vi "TFG.vi"() -> ()   [LabVIEW 2023]
uses:
  C:/Program Files (x86)/National Instruments/LabVIEW 2023/examples/Instrument IO/Serial/support/Serial - Settings.ctl
  <vilib>/Analysis/3filter.llb/Filter Passband Type.ctl
  <vilib>/Waveform/WDTOps.llb/WDT Waveform Duration DBL.vi
  <vilib>/Waveform/WDTOps.llb/WDT Number of Waveform Samples DBL.vi
  <vilib>/Waveform/WDTOps.llb/WDT Get Waveform Subset DBL.vi
  <vilib>/Analysis/3filter.llb/Butterworth Filter (DBL).vi
  <vilib>/measure/mamon.llb/Waveform Peak Detection for 1 Chan.vi
  <vilib>/express/express analysis/Spectral/Block/exnSpectralBlock spectral measurements power poly.vi
  <vilib>/express/express analysis/Spectral/Block/exnSpectralBlock spectral measurements power WFM.vi
  <vilib>/Instr/_visa.llb/VISA Configure Serial Port (Instr).vi
  <vilib>/express/express analysis/Spectral/XNode/ExpressSpectralMeasurementsBlockNode.xnode
  <vilib>/Analysis/NI_AALBase.lvlib
  <vilib>/measure/NI_MAPro.lvlib
  <vilib>/Analysis/NI_AALPro.lvlib
panel:
  in  "End Write on Termination Character? 2":bool=TRUE
  in  "Serial Settings (write) 2":T1={"baud rate"=9600, "data bits"=8, "parity"=enum."None", "stop bits"=10, "flow control"=0} {"flow control" items=["None"=0, "XON/XOFF"=1, "RTS/CTS"=2, "DTR/DSR"=4]; "stop bits" items=["1.0"=10, "1.5"=15, "2.0"=20]; "data bits" min=5 max=8 step=1; "baud rate" items=["75"=75, "110"=110, "134"=134, "150"=150, "300"=300, "600"=600, "1200"=1200, "1800"=1800, "2400"=2400, "4800"=4800, "7200"=7200, "9600"=9600, "14400"=14400, "19200"=19200, "28800"=28800, "38400"=38400, "56000"=56000, "57600"=57600, "115200"=115200, "128000"=128000, "230400"=230400]}
  in  "VISA Resource (write) 2":refnum<visa-resource-name>="COM1"
  out "bytes written 2":u32
  out "Formas de onda":waveform(dbl)[](graph)
  out "Señal Adquirida 2":waveform(dbl)[](graph)
  out "frecuencia manual 3":string
  out "frecuencia manual 1":string
  in  "banda 2":dbl
  in  "banda 1":dbl
  in  "peaks/valleys 2":u16(ring) items=["Peaks", "Valleys"]
  in  "duration":dbl=1.0 format="%0.2f"
  in  "alpha":dbl
  in  "path":path
  in  "Apagado":bool
  out "Baja con filtro":dbl
  out "baja sin filtro":dbl
  in  "Frecuencia manual1":dbl(slide) scale=150.0..3000.0
  in  "frecuencia manual 2":dbl(slide) scale=150.0..3000.0
  out "Espectro Amplitud":cluster{"f0":dbl, "df":dbl, "magnitude":dbl[]}(graph)
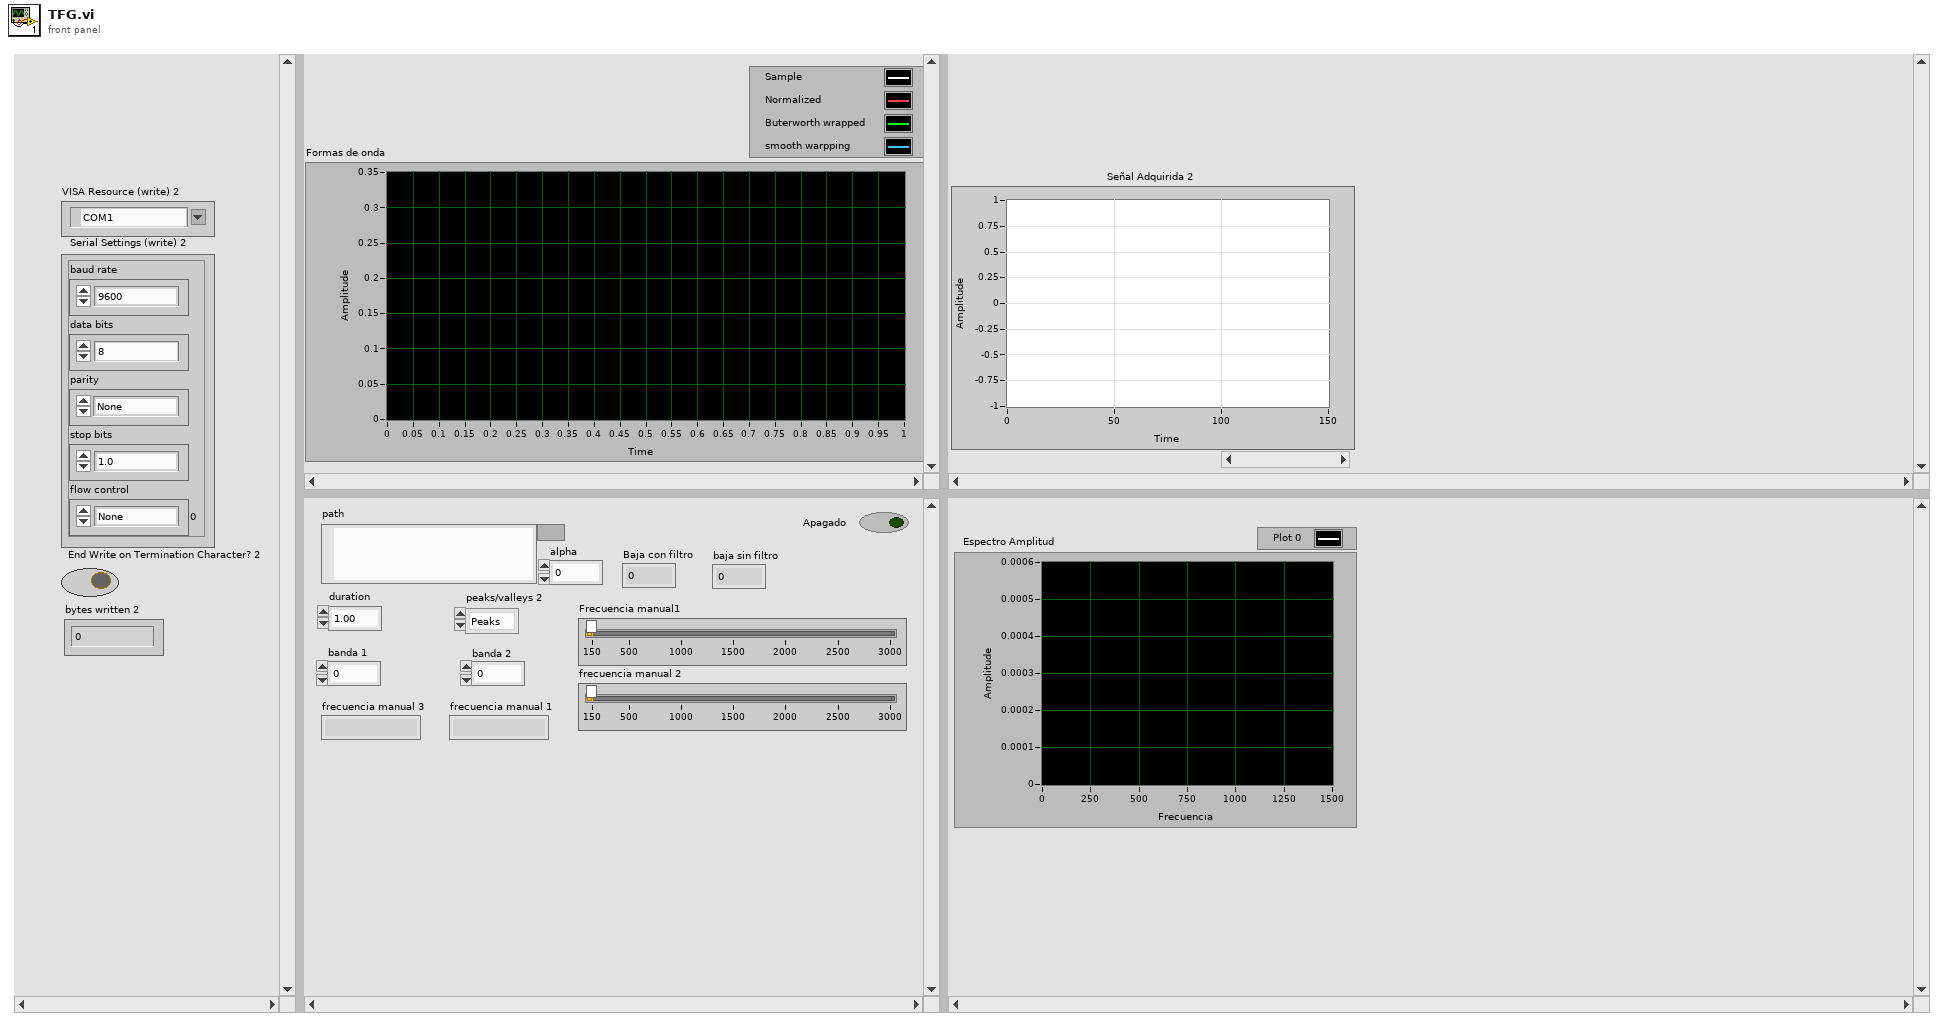
[diagram p1: front panel]
types:
  T1 = typedef "Serial - Settings.ctl" = cluster{"baud rate":u32, "data bits":u16, "parity":enum16{"None", "Odd", "Even", "Mark", "Space"}, "stop bits":u16, "flow control":u16}
  T2 = typedef "NI_AALBase.lvlib/Filter Passband Type.ctl" = enum32{"Lowpass", "Highpass", "Bandpass", "Bandstop"}
  T3 = cluster{"averaging mode":u16, "weighting mode":u16, "number of averages":u32}
  T4 = cluster{"dB On (F)":bool, "unwrap phase (F)":bool, "convert to degree (F)":bool}
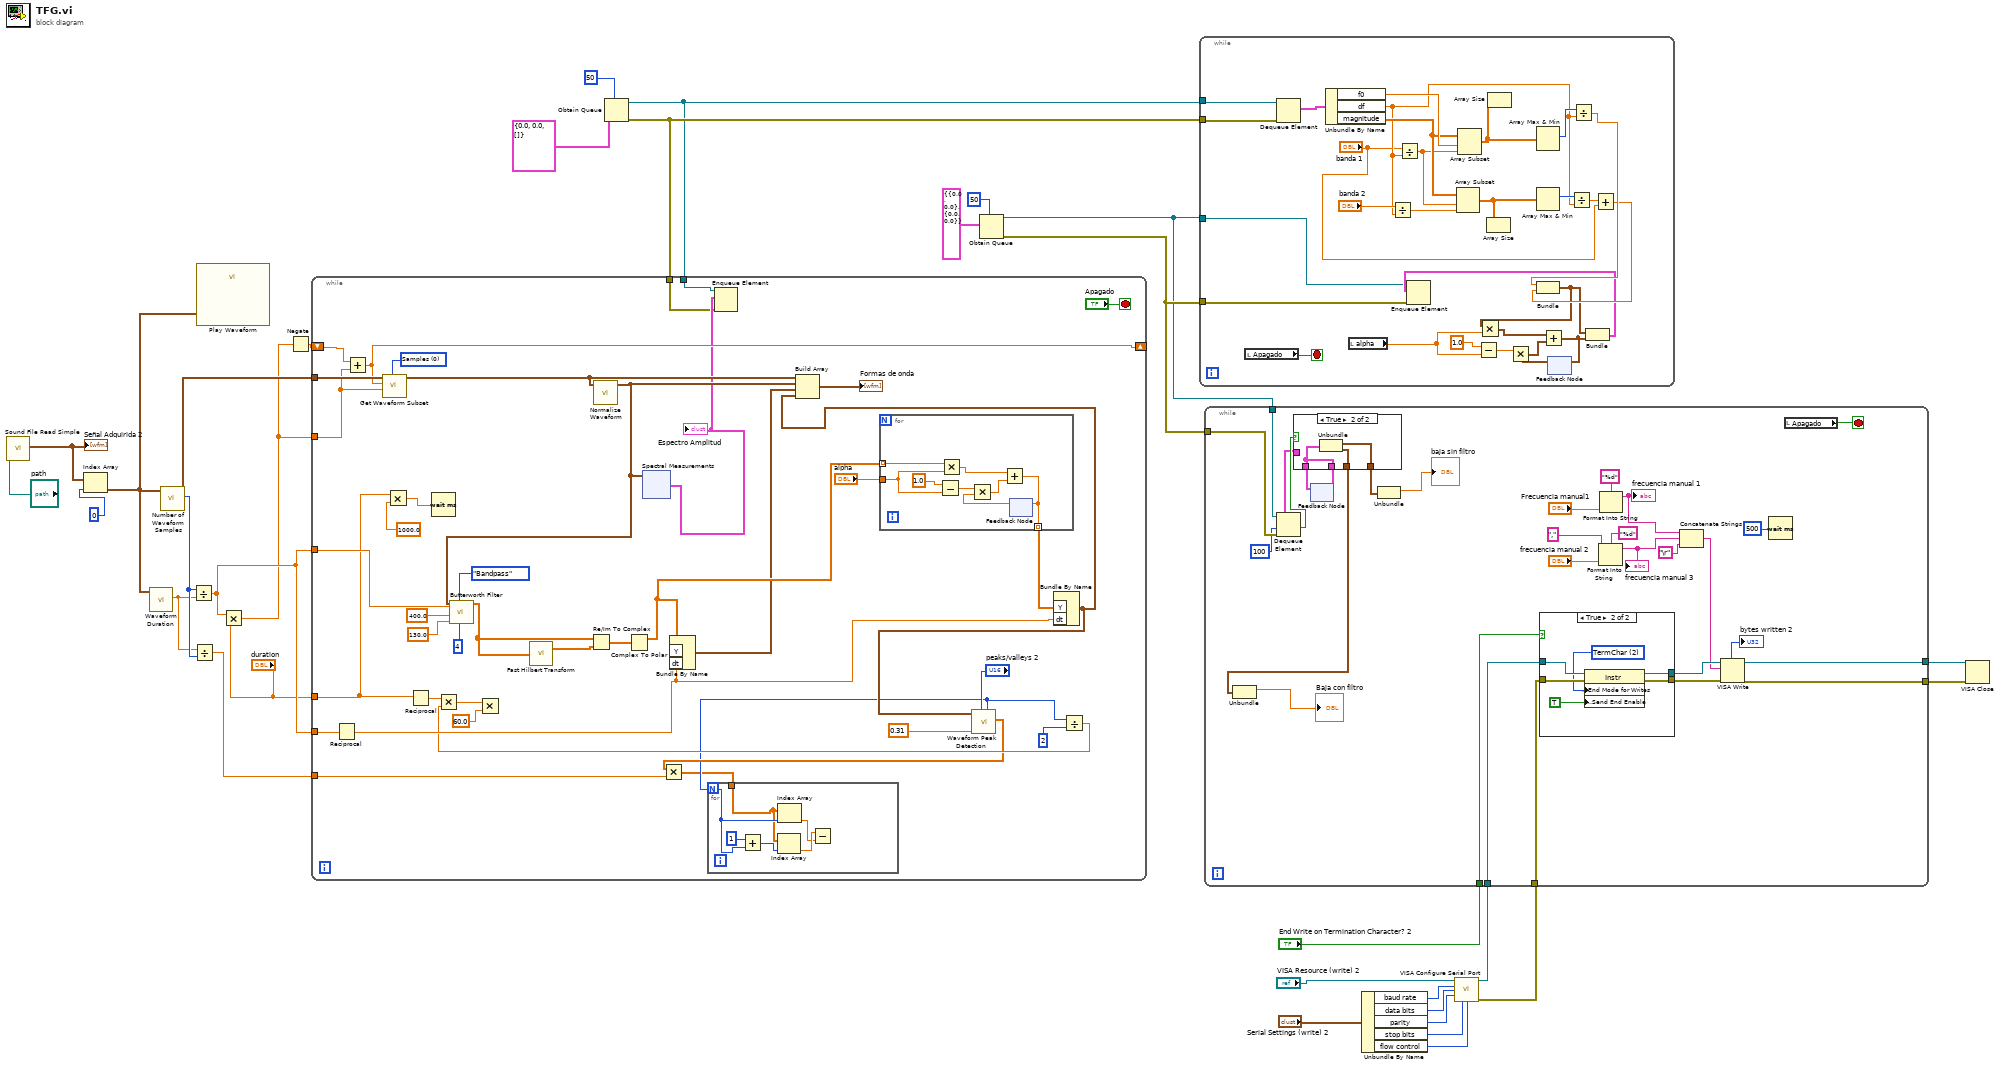
[diagram p0: block diagram]
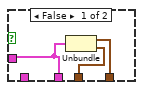
[diagram p3: hidden frame]
diagram:
  n1 = call <vilib>:"Sound File Read Simple.vi"("path"="path") -> ("data"=w31:waveform(dbl)[])  [unwired: 7 in, 3 out]
  "Señal Adquirida 2" <- w31
  n2 = Index Array(array=w31, index=0) -> (element=w22:waveform(dbl))
  n3 = call-poly <vilib>:"Waveform Duration.vi"("waveform in"=w22) -> ("duration"=w27:dbl)  [unwired: 8 in, 2 out]
  n4 = call-poly <vilib>:"Number of Waveform Samples.vi"("waveform in"=w22) -> ("number of samples"=w29:i32, "waveform out"=w28:waveform(dbl))  [unwired: 8 in, 1 out]
  n5 = Divide(x=w29, y=w27) -> (x/y=w25:dbl)
  n6 = Divide(x=w27, y=w29) -> (x/y=w26:dbl)
  n7 = call "Play Waveform"("Data"=w22) -> ()  [unwired: 18 in, 1 out]
  n8 = Multiply(x=w25, y="duration") -> (x*y=w24:dbl)
  n9 = Negate(x=w24) -> (-x=w23:dbl)
  n10 = Obtain Queue(max queue size (-1, unlimited)=50, element data type=cluster{"f0":dbl, "df":dbl, "magnitude":dbl[]} {"f0"=0.0, "df"=0.0, "magnitude"=[]} ("Power Spectrum")) -> (queue out=w16:refnum<queue>, error out=w19:errorcluster)  [unwired: 3 in, 1 out]
  n11 = while {
    tunnel: w28 -> [w47]
    tunnel: w26 -> [w46]
    tunnel: w25 -> [w45]
    shift-right: [w37] -> _
    shift-left: w23 -> [w38]
    tunnel: w25 -> [w41]
    tunnel: "duration" -> [w40]
    tunnel: w24 -> [w39]
    tunnel: w19 -> [w34]
    tunnel: w16 -> [w33]
    stop <- "Apagado" stop-if-true
    w42 = u16 0 items=["Samples", "Relative Time"] ("start/duration format")
    n12 = Reciprocal(x=w41) -> (1/x=w57:dbl)
    n13 = Add(x=w38, y=w39) -> (x+y=w37:dbl)
    n14 = call-poly <vilib>:"Get Waveform Subset.vi"("start/duration format"=w42, "duration"=w39, "start samples/time"=w37, "waveform in"=w47) -> ("waveform out"=w36:waveform(dbl))  [unwired: 2 in, 3 out]
    n15 = Multiply(x=w40, y=1000.0) -> (x*y=w44:dbl)
    n16 = Reciprocal(x=w40) -> (1/x=w54:dbl)
    n17 = Wait (ms)(milliseconds to wait=w44) -> ()  [unwired: 1 out]
    n18 = call <vilib>:"Normalize Waveform.vi"("waveform in"=w36) -> ("normalized waveform"=w68:waveform(dbl))  [unwired: 7 in, 3 out]
    n19 = call-poly <vilib>:"Butterworth Filter.vi"("order"=4, "filter type"=Filter_Passband_Type."Bandpass", "low cutoff freq: fl"=130.0, "high cutoff freq: fh"=400.0 ("low cutoff freq: fl"), "sampling freq: fs"=w45, "X"=w68) -> ("Filtered X"=w63:dbl[])  [unwired: 2 in, 1 out]
    n20 = call <vilib>:"Fast Hilbert Transform.vi"("X"=w63) -> ("Hilbert{X}"=w64:dbl[])  [unwired: 1 out]
    n21 = Re/Im To Complex(1:w64, 2:w63) -> (0:w62:cdb[])
    n22 = Complex To Polar(r * e^(i*theta)=w62) -> (r=w60:dbl[])  [unwired: 1 out]
    n23 = xnode "Spectral Measurements"("Signals"=w68) -> ("Power Spectrum"=w35:cluster{"f0":dbl, "df":dbl, "magnitude":dbl[]})  [unwired: 1 in, 1 out]
    "Espectro Amplitud" <- w35
    n24 = Bundle By Name("Y"=w60, "dt"=w57) -> (w48:waveform(dbl))  [unwired: 1 in]
    n25 = Enqueue Element(queue=w33, element=w35, error in (no error)=w34) -> ()  [unwired: 4 out]
    n26 = for {
      tunnel: "alpha" -> [w86]
      tunnel: w60 -> [w81] mode=indexing
      tunnel: [w80] -> w59 mode=indexing
      n27 = Subtract(x=1.0, y=w86) -> (x-y=w85:dbl)
      n28 = Multiply(x=w81, y=w86) -> (x*y=w83:dbl)
      n29 = feedback #1() -> (w82:dbl)  [unwired: 1 in]
      n30 = Multiply(x=w85, y=w82) -> (x*y=w84:dbl)
      n31 = Add(x=w83, y=w84) -> (x+y=w80:dbl)
      n32 = feedback-in #1(w80) -> ()
    }
    n33 = Bundle By Name("Y"=w59, "dt"=w57) -> (w58:waveform(dbl))  [unwired: 1 in]
    n34 = Build Array(w36, w68, w48, w58) -> (→"Formas de onda":waveform(dbl)[])
    n35 = call-poly <vilib>:"Waveform Peak Detection.vi"("peaks/valleys"="peaks/valleys 2", "threshold"=0.31, "Signal In"=w58) -> ("Locations"=w51:dbl[], "# found"=w50:i32)  [unwired: 4 in, 3 out]
    n36 = Multiply(x=w51, y=w46) -> (x*y=w49:dbl[])
    n37 = for {
      N: w50 -> [w77]
      tunnel: w49 -> [w76]
      n38 = Add(x=1 ("index"), y=w77) -> (x+y=w78:i32)
      n39 = Index Array(array=w76, index=w78) -> (element=w75:dbl)
      n40 = Index Array(array=w76, index=w77) -> (element=w74:dbl)
      n41 = Subtract(x=w75, y=w74) -> ()  [unwired: 1 out]
    }
    n42 = Divide(x=w50, y=2 ("threshold")) -> (x/y=w55:dbl)
    n43 = Multiply(x=w54, y=w55) -> (x*y=w53:dbl)
    n44 = Multiply(x=w53, y=60.0 ("low cutoff freq: fl")) -> ()  [unwired: 1 out]
  }
  n45 = Obtain Queue(max queue size (-1, unlimited)=50, element data type=cluster{cluster{dbl, dbl}, cluster{dbl, dbl}} {{0.0, 0.0}, {0.0, 0.0}} ("output cluster")) -> (queue out=w14:refnum<queue>, error out=w15:errorcluster)  [unwired: 3 in, 1 out]
  n46 = while {
    tunnel: w14 -> [w97]
    tunnel: w15 -> [w98]
    tunnel: w16 -> [w103]
    tunnel: w19 -> [w102]
    stop <- w99 stop-if-true
    n47 = local read "Apagado"() -> (w99:bool)
    n48 = Dequeue Element(queue=w103, error in (no error)=w102) -> (element=w101:cluster{"f0":dbl, "df":dbl, "magnitude":dbl[]})  [unwired: 4 out]
    n49 = Unbundle By Name(w101) -> ("f0"=w125:dbl, "df"=w115:dbl, "magnitude"=w123:dbl[])
    n50 = local read "alpha"() -> (w100:dbl)
    n51 = Divide(x="banda 2", y=w115) -> (x/y=w124:dbl)
    n52 = Divide(x="banda 1", y=w115) -> (x/y=w120:dbl)
    n53 = Array Subset(array=w123, index=w120, length=w124) -> (w119:dbl[])
    n54 = Array Subset(array=w123, index=w125, length=w120) -> (w121:dbl[])
    n55 = Subtract(x=1.0, y=w100) -> (x-y=w111:dbl)
    n56 = Array Size(array=w119) -> ()  [unwired: 1 out]
    n57 = Array Size(array=w121) -> ()  [unwired: 1 out]
    n58 = Array Max & Min(array=w121) -> (max index (indices)=w118:i32)  [unwired: 3 out]
    n59 = Array Max & Min(array=w119) -> (max index (indices)=w117:i32)  [unwired: 3 out]
    n60 = feedback #2() -> (w108:cluster{dbl, dbl})  [unwired: 1 in]
    n61 = Multiply(x=w111, y=w108) -> (x*y=w110:cluster{dbl, dbl})
    n62 = Divide(x=w117, y=w115) -> (x/y=w116:dbl)
    n63 = Divide(x=w118, y=w115) -> (x/y=w114:dbl)
    n64 = Add(x=w116, y="banda 1") -> (x+y=w113:dbl)
    n65 = Bundle(w114, w113) -> (w107:cluster{dbl, dbl})  [unwired: 1 in]
    n66 = Multiply(x=w107, y=w100) -> (x*y=w109:cluster{dbl, dbl})
    n67 = Add(x=w109, y=w110) -> (x+y=w106:cluster{dbl, dbl})
    n68 = feedback-in #2(w106) -> ()
    n69 = Bundle(w107, w106) -> (w105:cluster{cluster{dbl, dbl}, cluster{dbl, dbl}})  [unwired: 1 in]
    n70 = Enqueue Element(queue=w97, element=w105, error in (no error)=w98) -> ()  [unwired: 4 out]
  }
  n71 = Unbundle By Name("Serial Settings (write) 2") -> ("baud rate"=w10:u32, "data bits"=w9:u16, "parity"=w8:enum16{"None", "Odd", "Even", "Mark", "Space"}, "stop bits"=w7:u16, "flow control"=w6:u16)
  n72 = call-poly "VISA Configure Serial Port"("VISA resource name"="VISA Resource (write) 2", "baud rate (9600)"=w10, "data bits (8)"=w9, "parity (0:none)"=w8, "stop bits (10: 1 bit)"=w7, "flow control (0:none)"=w6) -> ("VISA resource name out"=w3:refnum<visa-resource-name>, "error out"=w4:errorcluster)  [unwired: 3 in, 5 out]
  n73 = while {
    tunnel: w14 -> [w155]
    tunnel: w15 -> [w154]
    tunnel: "End Write on Termination Character? 2" -> [w129]
    tunnel: w4 -> [w130]
    tunnel: w3 -> [w128]
    tunnel: [w127] -> w2
    tunnel: [w126] -> w1
    stop <- w147 stop-if-true
    n74 = Dequeue Element(queue=w155, timeout in ms (-1)=100, error in (no error)=w154) -> (element=w149:cluster{cluster{dbl, dbl}, cluster{dbl, dbl}}, timed out?=w152:bool)  [unwired: 2 out]
    n75 = feedback #3() -> (w150:cluster{cluster{dbl, dbl}, cluster{dbl, dbl}})  [unwired: 1 in]
    n76 = case shown="True" w152 {
      tunnel: [w166 w169] -> w146
      tunnel: [w165 w168] -> w151
      tunnel: w150 -> [_ w167]
      tunnel: w149 -> [w164 _]
      tunnel: [w164 w167] -> w148
      frame False {
        n77 = Unbundle(w164) -> (w166:cluster{dbl, dbl}, w165:cluster{dbl, dbl})
      }
      frame True {
        n78 = Unbundle(w167) -> (w169:cluster{dbl, dbl}, w168:cluster{dbl, dbl})
      }
    }
    n79 = Unbundle(w151) -> (→"Baja con filtro":dbl)  [unwired: 1 out]
    n80 = feedback-in #3(w148) -> ()
    n81 = Unbundle(w146) -> (→"baja sin filtro":dbl)  [unwired: 1 out]
    n82 = case shown="True" w129 {
      tunnel: w128 -> [w156 w163]
      tunnel: w130 -> [w157 w162]
      tunnel: [w156 w161] -> w143
      tunnel: [w157 w160] -> w142
      frame False {
      }
      frame True {
        w159 = u16 2 items=["None", "LastBit", "TermChar", "Break"] ("Serial Settings:Serial End Mode for Writes")
        n83 = property class="Instr"(reference=w163, error in=w162, "Serial Settings:End Mode for Writes"=w159, "Message Based Settings:Send End Enable"=TRUE) -> (reference out=w161:refnum<visa-resource-name>, error out=w160:errorcluster)
      }
    }
    n84 = Format Into String(format string="%d", initial string=",", "frecuencia manual 2") -> (resulting string=w134:string)  [unwired: 1 in, 1 out]
    "frecuencia manual 3" <- w134
    n85 = Format Into String(format string="%d", "Frecuencia manual1") -> (resulting string=w135:string)  [unwired: 2 in, 1 out]
    "frecuencia manual 1" <- w135
    n86 = Concatenate Strings(w135, w134, "\r") -> (w141:string)
    n87 = VISA Write(VISA resource name=w143, write buffer=w141, error in (no error)=w142) -> (VISA resource name out=w127:refnum<visa-resource-name>, return count=→"bytes written 2":u32, error out=w126:errorcluster)
    n88 = Wait (ms)(milliseconds to wait=u32 500) -> ()  [unwired: 1 out]
    n89 = local read "Apagado"() -> (w147:bool)
  }
  n90 = VISA Close(VISA resource name=w2, error in (no error)=w1) -> ()  [unwired: 1 out]
